vi "AT Is Enum Index Available A.vi"(8 "error in (no error)":errorcluster, 9 "Index":i32, 10 "Feature":string, 11 "Handle":i32) -> (0 "error out":errorcluster, 2 "Available":bool, 3 "Status":i32)   [LabVIEW 2019]
doc: "Is Enum Index Available\n\nOutput:\n I32 Status\n Bool Available\n\nInput:\n I32 Handle\n String Feature\n I32 Index\n\nThis function indicates whether the specified enumerated feature index can currently be selected. The\navailability of enumerated options may depend on the value of other features."
uses:
  atcoreA.dll
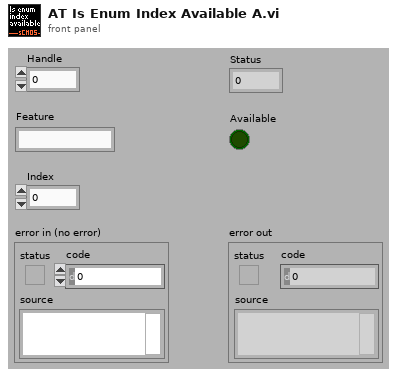
[diagram p1: front panel]
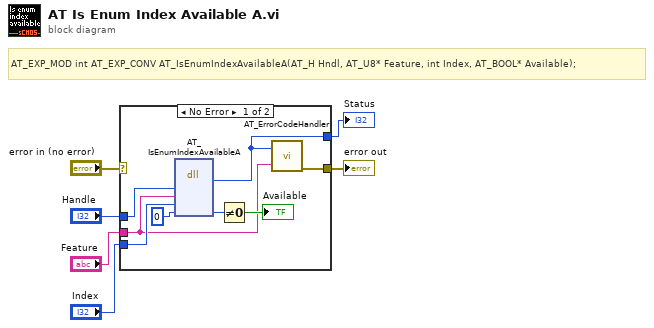
[diagram p0: block diagram]
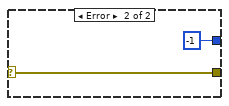
[diagram p2: hidden frame]
diagram:
  # "AT_EXP_MOD int AT_EXP_CONV AT_IsEnumIndexAvailableA(AT_H Hndl, AT_U8* Feature, int Index, AT_BOOL* Available);"
  n1 = case shown="No Error" "error in (no error)" {
    selector: "error in (no error)" -> [_ w16]
    tunnel: [w8 -1] -> w6
    tunnel: "Handle" -> [w14 _]
    tunnel: "Feature" -> [w7 _]
    tunnel: "Index" -> [w13 _]
    tunnel: [w9 w16] -> w1
    frame No Error {
      n2 = dll-call lib="atcoreA.dll" fn="AT_IsEnumIndexAvailableA"("Handle"=w14, "Feature"=w7, "Index"=w13, "Available"=0) -> ("Status"=w8:i32, "Available"=w10:i32)  [unwired: 6 in, 2 out]
      n3 = Not Equal To 0?(x=w10) -> (x != 0?=→"Available":bool)
      n4 = call <userlib>:"AT_ErrorCodeHandler.vi"("Error"=w8, "Feature Name"=w7) -> ("error out"=w9:errorcluster)  [unwired: 5 in]
    }
    frame Error {
    }
  }
  "Status" <- w6
  "error out" <- w1
